vi "in_spline system y1.vi"(4 "final boundary":T1, 6 "initial boundary":T1, 10 "X":dbl[](array[numeric]), 11 "Y":dbl[](array[numeric])) -> (2 "b":dbl[](array[numeric]), 3 "A":T2)   [LabVIEW 2024, in "NI_Gmath.lvlib"]
uses:
  NI_Gmath.lvlib
  RealMatrix.ctl
  in_diff and divided diff (dy over dx).vi
  in_diff and divided diff (dx).vi
  Array To Matrix - RA2.vi
  NI_Matrix.lvlib
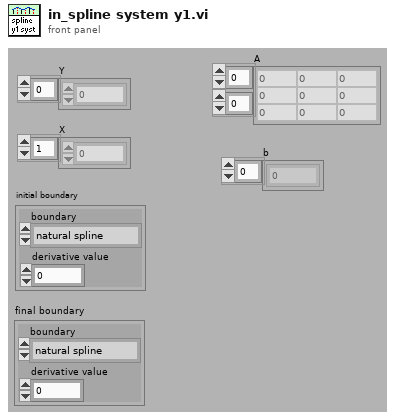
[diagram p1: front panel]
types:
  T1 = cluster{"boundary":enum16{"natural spline", "not-a-knot", "1st derivative", "2nd derivative"}, "derivative value":dbl}
  T2 = typedef "NI_Matrix.lvlib/RealMatrix.ctl" = dbl[][]
  T3 = enum16{"natural spline", "not-a-knot", "1st derivative", "2nd derivative"}
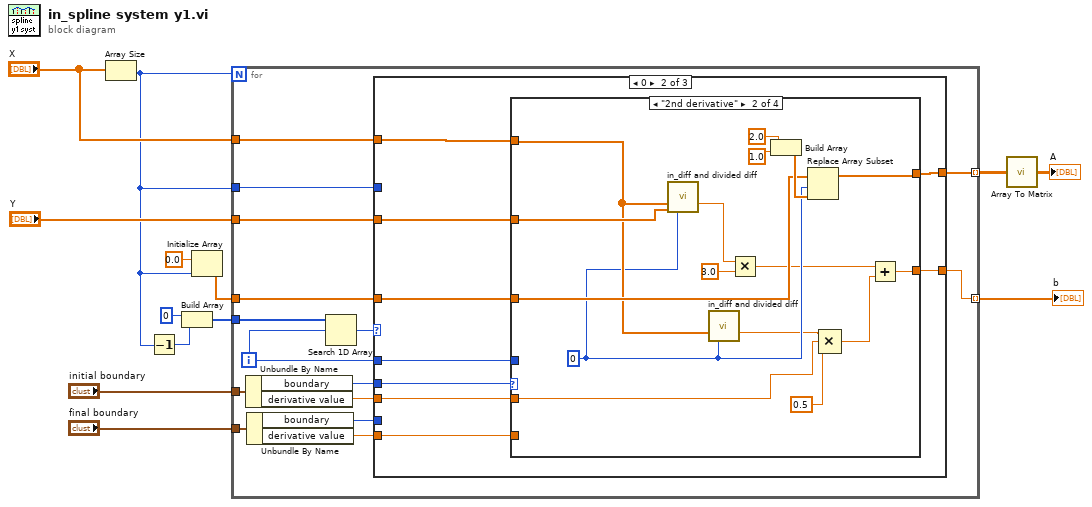
[diagram p0: block diagram]
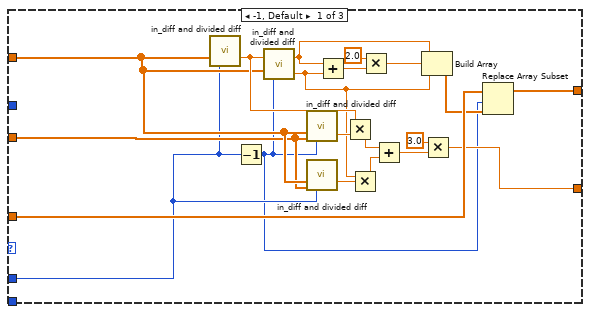
[diagram p2: hidden frame]
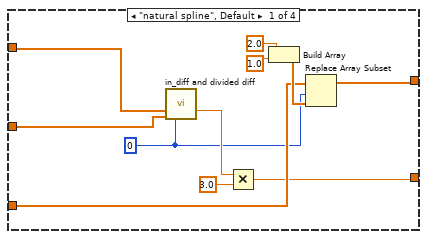
[diagram p3: hidden frame]
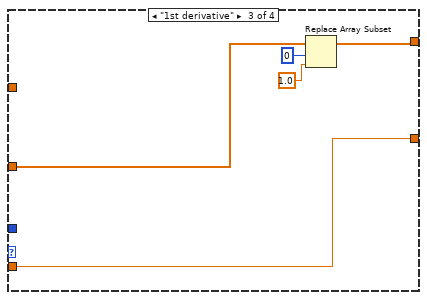
[diagram p4: hidden frame]
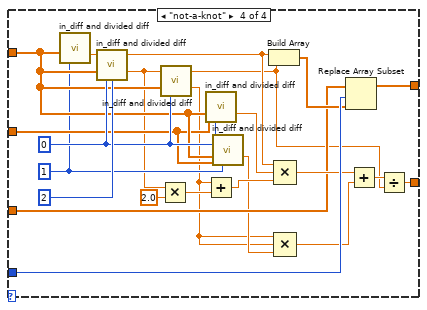
[diagram p5: hidden frame]
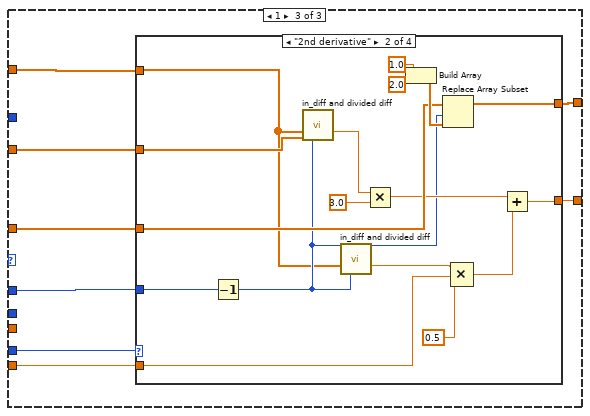
[diagram p6: hidden frame]
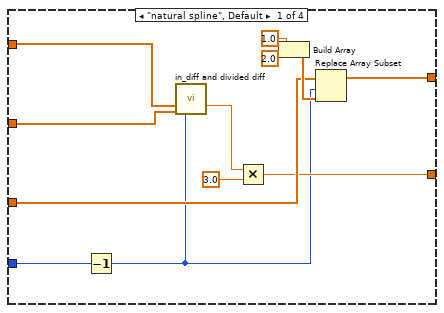
[diagram p7: hidden frame]
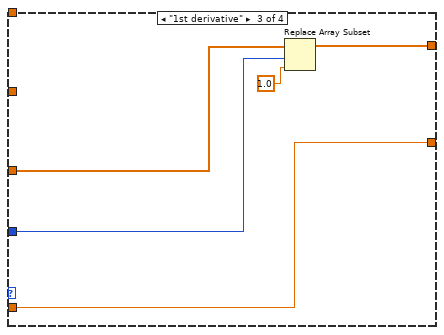
[diagram p8: hidden frame]
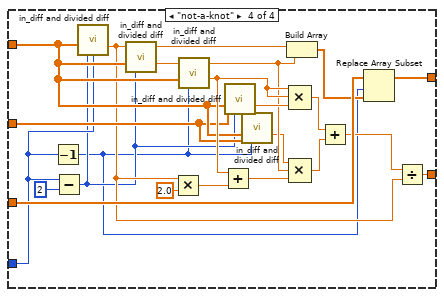
[diagram p9: hidden frame]
diagram:
  n1 = Array Size(array="X") -> (size(s)=w9:i32)
  n2 = Decrement(x=w9) -> (x-1=w7:i32)
  n3 = Build Array(0 ("element"), w7) -> (w8:i32[])
  n4 = Initialize Array(0.0 ("element"), w9) -> (w5:dbl[])
  n5 = for {
    N: w9 -> [_]
    tunnel: "X" -> [w28]
    tunnel: "Y" -> [w27]
    tunnel: w5 -> [w26]
    tunnel: [w25] -> w10 mode=indexing
    tunnel: w8 -> [w24]
    tunnel: [w21] -> w11 mode=indexing
    tunnel: w9 -> [w20]
    tunnel: "initial boundary" -> [w19]
    tunnel: "final boundary" -> [w18]
    i -> [w22]
    n6 = Unbundle By Name(w19) -> ("boundary"=w17:T3, "derivative value"=w14:dbl)
    n7 = Unbundle By Name(w18) -> ("boundary"=w16:T3, "derivative value"=w15:dbl)
    n8 = Search 1D Array(1D array=w24, element=w22) -> (index of element=w23:i32)  [unwired: 1 in]
    n9 = case shown="0" w23 {
      tunnel: w28 -> [w35 w52 w114]
      tunnel: w27 -> [w34 w51 w113]
      tunnel: w26 -> [w46 w53 w117]
      tunnel: w22 -> [w30 w54 w112]
      tunnel: [w43 w56 w116] -> w25
      tunnel: [w41 w55 w115] -> w21
      tunnel: w20 -> [_ _ _]
      tunnel: w17 -> [_ w50 _]
      tunnel: w16 -> [_ _ w111]
      tunnel: w15 -> [_ w48 w110]
      tunnel: w14 -> [_ w49 _]
      frame -1, Default {
        n10 = call-poly "in_diff and divided diff.vi"("X"=w35, "i1"=w30) -> ("difference"=w36:dbl)  [unwired: 13 in]
        n11 = Decrement(x=w30) -> (x-1=w29:i32)
        n12 = call-poly "in_diff and divided diff.vi"("X"=w35, "i1"=w29) -> ("difference"=w32:dbl)  [unwired: 13 in]
        n13 = call-poly "in_diff and divided diff.vi"("X"=w35, "Y"=w34, "i1"=w29) -> ("difference"=w37:dbl)  [unwired: 12 in]
        n14 = call-poly "in_diff and divided diff.vi"("X"=w35, "Y"=w34, "i1"=w30) -> ("difference"=w33:dbl)  [unwired: 12 in]
        n15 = Add(x=w36, y=w32) -> (x+y=w40:dbl)
        n16 = Multiply(x=w36, y=w37) -> (x*y=w39:dbl)
        n17 = Multiply(x=w32, y=w33) -> (x*y=w31:dbl)
        n18 = Multiply(x=2.0, y=w40) -> (x*y=w45:dbl)
        n19 = Add(x=w39, y=w31) -> (x+y=w38:dbl)
        n20 = Build Array(w36, w45, w32) -> (w44:dbl[])
        n21 = Multiply(x=3.0, y=w38) -> (x*y=w41:dbl)
        n22 = Replace Array Subset(array=w46, new element=w44, index=w29) -> (w43:dbl[])
      }
      frame 0 {
        n23 = case shown="\"2nd derivative\"" w50 {
          tunnel: [w62 w78 w88 w109] -> w56
          tunnel: [w58 w69 w84 w105] -> w55
          tunnel: w54 -> [_ _ _ w104]
          tunnel: w53 -> [w59 w76 w87 w95]
          tunnel: w52 -> [w61 w75 _ w94]
          tunnel: w51 -> [w60 w77 _ w93]
          tunnel: w49 -> [_ w68 w84 _]
          tunnel: w48 -> [_ _ _ _]
          frame "natural spline", Default {
            w57 = 0 ("x+1")
            n24 = call-poly "in_diff and divided diff.vi"("X"=w61, "Y"=w60, "i1"=w57) -> ("difference"=w63:dbl)  [unwired: 12 in]
            n25 = Multiply(x=w63, y=3.0 ("x")) -> (x*y=w58:dbl)
            n26 = Build Array(2.0, 1.0) -> (w66:dbl[])
            n27 = Replace Array Subset(array=w59, new element=w66, index=w57) -> (w62:dbl[])
          }
          frame "2nd derivative" {
            w74 = 0 ("x+1")
            n28 = call-poly "in_diff and divided diff.vi"("X"=w75, "Y"=w77, "i1"=w74) -> ("difference"=w79:dbl)  [unwired: 12 in]
            n29 = call-poly "in_diff and divided diff.vi"("X"=w75, "i1"=w74) -> ("difference"=w73:dbl)  [unwired: 13 in]
            n30 = Multiply(x=w79, y=3.0 ("x")) -> (x*y=w71:dbl)
            n31 = Build Array(2.0, 1.0) -> (w82:dbl[])
            n32 = Replace Array Subset(array=w76, new element=w82, index=w74) -> (w78:dbl[])
            n33 = Compound Arithmetic op=MULTIPLY(w73, w68, 0.5 ("value")) -> (w70:dbl)
            n34 = Add(x=w71, y=w70) -> (x+y=w69:dbl)
          }
          frame "1st derivative" {
            n35 = Replace Array Subset(array=w87, new element=1.0, index=0 ("x+1")) -> (w88:dbl[])
          }
          frame "not-a-knot" {
            w96 = 0 ("x+1")
            w92 = 1 ("x+1")
            n36 = call-poly "in_diff and divided diff.vi"("X"=w94, "i1"=w92) -> ("difference"=w98:dbl)  [unwired: 13 in]
            n37 = call-poly "in_diff and divided diff.vi"("X"=w94, "i1"=w96, "i2"=2 ("x+1")) -> ("difference"=w90:dbl)  [unwired: 12 in]
            n38 = Multiply(x=w90, y=2.0 ("x")) -> (x*y=w107:dbl)
            n39 = call-poly "in_diff and divided diff.vi"("X"=w94, "i1"=w96) -> ("difference"=w89:dbl)  [unwired: 13 in]
            n40 = call-poly "in_diff and divided diff.vi"("X"=w94, "Y"=w93, "i1"=w96) -> ("difference"=w97:dbl)  [unwired: 12 in]
            n41 = Add(x=w89, y=w107) -> (x+y=w101:dbl)
            n42 = call-poly "in_diff and divided diff.vi"("X"=w94, "Y"=w93, "i1"=w92) -> ("difference"=w91:dbl)  [unwired: 12 in]
            n43 = Build Array(w98, w90) -> (w100:dbl[])
            n44 = Compound Arithmetic op=MULTIPLY(w98, w97, w101) -> (w99:dbl)
            n45 = Compound Arithmetic op=MULTIPLY(w89, w89, w91) -> (w102:dbl)
            n46 = Replace Array Subset(array=w95, new element=w100, index=w104) -> (w109:dbl[])
            n47 = Add(x=w99, y=w102) -> (x+y=w106:dbl)
            n48 = Divide(x=w106, y=w90) -> (x/y=w105:dbl)
          }
        }
      }
      frame 1 {
        n49 = case shown="\"2nd derivative\"" w111 {
          tunnel: w117 -> [w121 w139 w148 w172]
          tunnel: [w124 w141 w150 w171] -> w116
          tunnel: [w120 w134 w147 w170] -> w115
          tunnel: w114 -> [w123 w131 _ w161]
          tunnel: w113 -> [w122 w140 _ w160]
          tunnel: w112 -> [w119 w138 w149 w155]
          tunnel: w110 -> [_ w130 w147 _]
          frame "natural spline", Default {
            n50 = Decrement(x=w119) -> (x-1=w118:i32)
            n51 = call-poly "in_diff and divided diff.vi"("X"=w123, "Y"=w122, "i1"=w118) -> ("difference"=w125:dbl)  [unwired: 12 in]
            n52 = Multiply(x=w125, y=3.0 ("x")) -> (x*y=w120:dbl)
            n53 = Build Array(1.0, 2.0) -> (w128:dbl[])
            n54 = Replace Array Subset(array=w121, new element=w128, index=w118) -> (w124:dbl[])
          }
          frame "2nd derivative" {
            n55 = Decrement(x=w138) -> (x-1=w132:i32)
            n56 = call-poly "in_diff and divided diff.vi"("X"=w131, "Y"=w140, "i1"=w132) -> ("difference"=w142:dbl)  [unwired: 12 in]
            n57 = call-poly "in_diff and divided diff.vi"("X"=w131, "i1"=w132) -> ("difference"=w137:dbl)  [unwired: 13 in]
            n58 = Multiply(x=w142, y=3.0 ("x")) -> (x*y=w135:dbl)
            n59 = Build Array(1.0, 2.0) -> (w145:dbl[])
            n60 = Replace Array Subset(array=w139, new element=w145, index=w132) -> (w141:dbl[])
            n61 = Compound Arithmetic op=MULTIPLY(w137, w130, 0.5 ("value")) -> (w133:dbl)
            n62 = Add(x=w135, y=w133) -> (x+y=w134:dbl)
          }
          frame "1st derivative" {
            n63 = Replace Array Subset(array=w148, new element=1.0, index=w149) -> (w150:dbl[])
          }
          frame "not-a-knot" {
            n64 = Decrement(x=w155) -> (x-1=w152:i32)
            n65 = Subtract(x=w155, y=2) -> (x-y=w153:i32)
            n66 = call-poly "in_diff and divided diff.vi"("X"=w161, "i1"=w153, "i2"=w155) -> ("difference"=w154:dbl)  [unwired: 12 in]
            n67 = call-poly "in_diff and divided diff.vi"("X"=w161, "i1"=w153) -> ("difference"=w162:dbl)  [unwired: 13 in]
            n68 = Multiply(x=w154, y=2.0) -> (x*y=w165:dbl)
            n69 = call-poly "in_diff and divided diff.vi"("X"=w161, "i1"=w152) -> ("difference"=w164:dbl)  [unwired: 13 in]
            n70 = Add(x=w164, y=w165) -> (x+y=w163:dbl)
            n71 = call-poly "in_diff and divided diff.vi"("X"=w161, "Y"=w160, "i1"=w153) -> ("difference"=w167:dbl)  [unwired: 12 in]
            n72 = call-poly "in_diff and divided diff.vi"("X"=w161, "Y"=w160, "i1"=w152) -> ("difference"=w159:dbl)  [unwired: 12 in]
            n73 = Build Array(w154, w162) -> (w168:dbl[])
            n74 = Compound Arithmetic op=MULTIPLY(w164, w164, w167) -> (w157:dbl)
            n75 = Compound Arithmetic op=MULTIPLY(w159, w162, w163) -> (w158:dbl)
            n76 = Add(x=w157, y=w158) -> (x+y=w156:dbl)
            n77 = Replace Array Subset(array=w172, new element=w168, index=w152) -> (w171:dbl[])
            n78 = Divide(x=w156, y=w154) -> (x/y=w170:dbl)
          }
        }
      }
    }
  }
  "b" <- w11
  n79 = call-poly "Array To Matrix.vi"("Real 2D Array"=w10) -> ("Real Matrix"=→"A":T2)
